vi "fgv_Enforce AOL Z repeat.vi"(8 "error in (no error)":errorcluster, 9 "Function":T1, 11 "Enforce AOL Z repeat":bool) -> (0 "error out":errorcluster, 3 "Enforce AOL Z repeat?":bool)   [LabVIEW 2017]
uses:
  Typedefs/Read Write Enum.ctl
panel:
  # "SUBROUTINE"
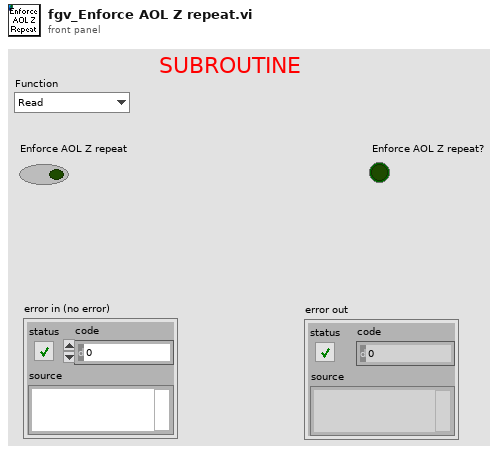
[diagram p1: front panel]
types:
  T1 = typedef "Read Write Enum.ctl" = enum16{"Read", "Write"}
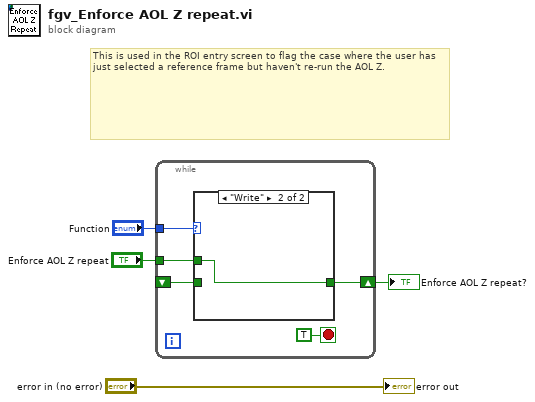
[diagram p0: block diagram]
diagram:
  # "This is used in the ROI entry screen to flag the case where the user has just selected a reference frame but haven't re-run the AOL Z."
  n1 = while {
    tunnel: "Function" -> [w8]
    tunnel: "Enforce AOL Z repeat" -> [w7]
    shift-right: [w6] -> w2
    shift-left: _ -> [w5]
    stop <- TRUE stop-if-true
    n2 = case shown="\"Write\"" w8 {
      tunnel: w7 -> [_ w11]
      tunnel: [w10 w11] -> w6
      tunnel: w5 -> [w10 _]
      frame "Read", Default {
      }
      frame "Write" {
      }
    }
  }
  "Enforce AOL Z repeat?" <- w2
  "error out" <- "error in (no error)"
